vi "Write Error Log.vi"(8 "Byte Stream File in":refnum<file>, 11 "error in (no error)":errorcluster) -> ()   [LabVIEW 2016]
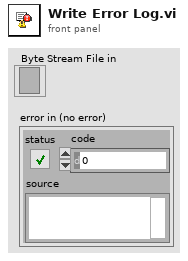
[diagram p1: front panel]
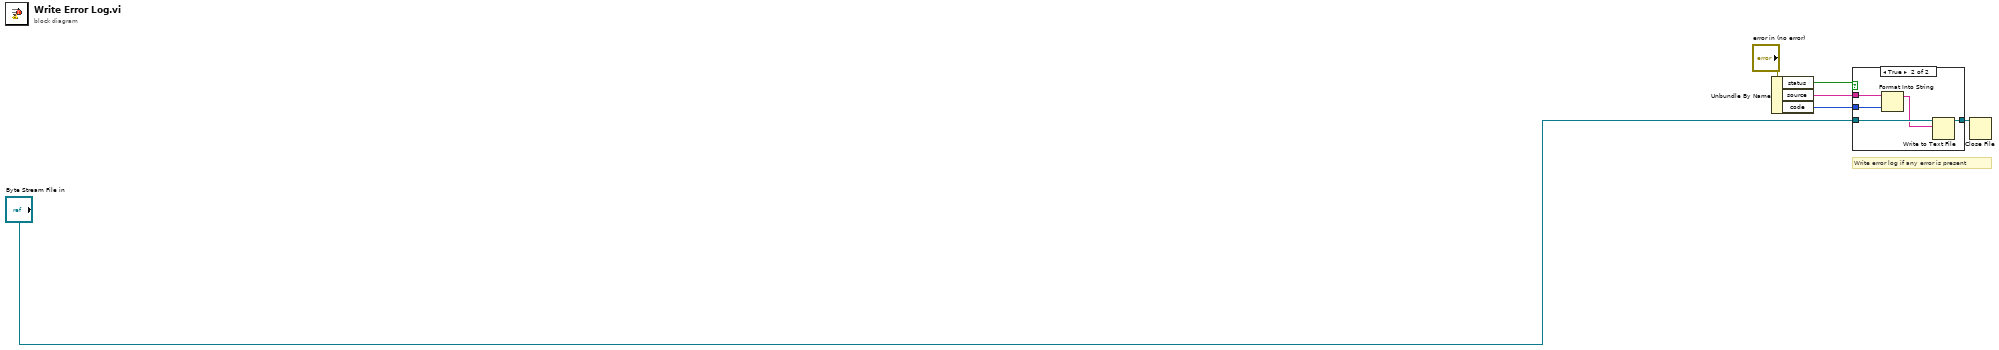
[diagram p0: block diagram]
diagram:
  # "Write error log if any error is present"
  n1 = Unbundle By Name("error in (no error)") -> ("status"=w2:bool, "source"=w4:string, "code"=w5:i32)
  n2 = case shown="True" w2 {
    tunnel: "Byte Stream File in" -> [w7 w12]
    tunnel: w4 -> [_ w10]
    tunnel: w5 -> [_ w9]
    tunnel: [w7 w8] -> w6
    frame False {
    }
    frame True {
      n3 = Format Into String(initial string=w10, w9) -> (resulting string=w11:string)  [unwired: 2 in, 1 out]
      n4 = Write to Text File(file (use dialog)=w12, text=w11) -> (refnum out=w8:refnum<file>)  [unwired: 2 in, 2 out]
    }
  }
  n5 = Close File(refnum=w6) -> ()  [unwired: 1 in, 2 out]
